vi "Logging Unflatten.vi"(1 "In":T4) -> (0 "Out":T1)   [LabVIEW 2012, in "femtoRoboLib.lvlib"]
uses:
  femtoRoboLib.lvlib
  Controls/Log Entry - Converted.ctl
  Controls/Log Entry.ctl
  Controls/Log Value Type.ctl
  Controls/Log Value Cluster.ctl
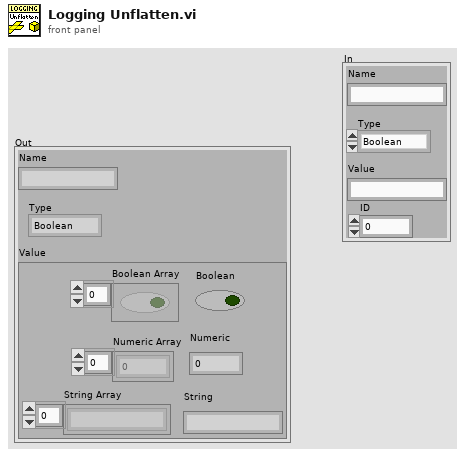
[diagram p1: front panel]
types:
  T1 = typedef "femtoRoboLib.lvlib/Log Entry.ctl" = cluster{"Name":string, "Type":T2, "Value":T3}
  T2 = typedef "femtoRoboLib.lvlib/Log Value Type.ctl" = enum16{"Boolean", "Numeric", "String", "Boolean Array", "Numeric Array", "String Array"}
  T3 = typedef "femtoRoboLib.lvlib/Log Value Cluster.ctl" = cluster{"Boolean Array":bool[], "Boolean":bool, "Numeric Array":dbl[], "Numeric":dbl, "String Array":string[], "String":string}
  T4 = typedef "femtoRoboLib.lvlib/Log Entry - Converted.ctl" = cluster{"Name":string, "Type":enum16{"Boolean", "Numeric", "String", "Boolean Array", "Numeric Array", "String Array"}, "Value":string, "ID":u32}
  T5 = enum16{"Boolean", "Numeric", "String", "Boolean Array", "Numeric Array", "String Array"}
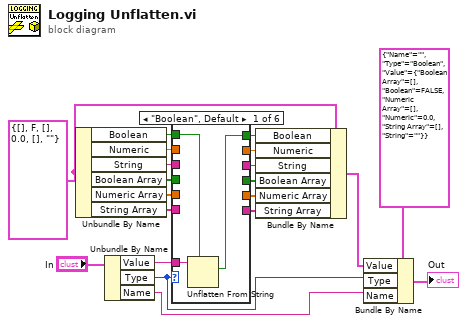
[diagram p0: block diagram]
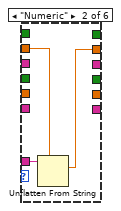
[diagram p2: hidden frame]
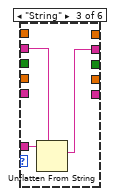
[diagram p3: hidden frame]
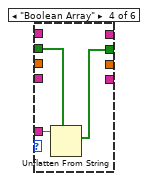
[diagram p4: hidden frame]
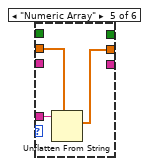
[diagram p5: hidden frame]
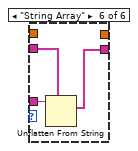
[diagram p6: hidden frame]
diagram:
  w12 = T3 {"Boolean Array"=[], "Boolean"=FALSE, "Numeric Array"=[], "Numeric"=0.0, "String Array"=[], "String"=""} ("Log Value Cluster")
  n1 = Unbundle By Name(w12) -> ("Boolean"=w19:bool, "Numeric"=w18:dbl, "String"=w17:string, "Boolean Array"=w16:bool[], "Numeric Array"=w15:dbl[], "String Array"=w14:string[])
  n2 = Unbundle By Name("In") -> ("Value"=w13:string, "Type"=w3:T5, "Name"=w2:string)
  n3 = case shown="\"Boolean\", Default" w3 {
    tunnel: w19 -> [w23 _ _ _ _ _]
    tunnel: w18 -> [_ w26 _ _ _ _]
    tunnel: w17 -> [_ _ w28 _ _ _]
    tunnel: w16 -> [_ _ _ w30 _ _]
    tunnel: w15 -> [_ _ _ _ w34 _]
    tunnel: w14 -> [_ _ _ _ _ w38]
    tunnel: w13 -> [w22 w25 w29 w32 w35 w37]
    tunnel: [w21 _ _ _ _ _] -> w11
    tunnel: [_ w24 _ _ _ _] -> w10
    tunnel: [_ _ w27 _ _ _] -> w9
    tunnel: [_ _ _ w31 _ _] -> w8
    tunnel: [_ _ _ _ w33 _] -> w7
    tunnel: [_ _ _ _ _ w36] -> w6
    frame "Boolean", Default {
      n4 = Unflatten From String(type=w23, binary string=w22) -> (value=w21:bool)  [unwired: 3 in, 2 out]
    }
    frame "Numeric" {
      n5 = Unflatten From String(type=w26, binary string=w25) -> (value=w24:dbl)  [unwired: 3 in, 2 out]
    }
    frame "String" {
      n6 = Unflatten From String(type=w28, binary string=w29) -> (value=w27:string)  [unwired: 3 in, 2 out]
    }
    frame "Boolean Array" {
      n7 = Unflatten From String(type=w30, binary string=w32) -> (value=w31:bool[])  [unwired: 3 in, 2 out]
    }
    frame "Numeric Array" {
      n8 = Unflatten From String(type=w34, binary string=w35) -> (value=w33:dbl[])  [unwired: 3 in, 2 out]
    }
    frame "String Array" {
      n9 = Unflatten From String(type=w38, binary string=w37) -> (value=w36:string[])  [unwired: 3 in, 2 out]
    }
  }
  n10 = Bundle By Name(cluster=w12, "Boolean"=w11, "Numeric"=w10, "String"=w9, "Boolean Array"=w8, "Numeric Array"=w7, "String Array"=w6) -> (w4:T3)
  n11 = Bundle By Name(cluster=T1 {"Name"="", "Type"=enum."Boolean", "Value"={"Boolean Array"=[], "Boolean"=FALSE, "Numeric Array"=[], "Numeric"=0.0, "String Array"=[], "String"=""}} ("Log Variable"), "Value"=w4, "Type"=w3, "Name"=w2) -> (→"Out":T1)
